vi "RPC Method MeasurementService Measure Logic.vi"(8 "error in":errorcluster, 11 "gRPCid in":T1) -> (0 "error out":errorcluster)   [LabVIEW 2020, in "MeasurementLink Measurement Server.lvlib"]
uses:
  MeasurementLink Measurement Server.lvlib
  <vilib>/gRPC/LabVIEW gRPC Library/Shared/grpcId.ctl
  Measurement Configuration.ctl
  <vilib>/gRPC/LabVIEW gRPC Library/Server API/typeDefs/gRPC Status Code.ctl
  6e93e594-9b53-4a41-bad0-565312cbf1e4.vi
  c01dd925-8d21-4ce6-b452-e7218c44af5c.vi
  <vilib>/gRPC/LabVIEW gRPC Library/Server API/Translate Protobuf Error.vi
  <vilib>/AdvancedString/1D String Array to Delimited String.vi
  <vilib>/gRPC/LabVIEW gRPC Library/Server API/Server/Get Server DLL Path.vi
  MeasurementContext/MeasurementContext.lvclass
  <vilib>/gRPC/LabVIEW gRPC Library/grpc-lvsupport-release.lvlib
  MeasurementLink Measurement Server Internal/RPC Service/MeasurementService/MeasurementService.lvclass
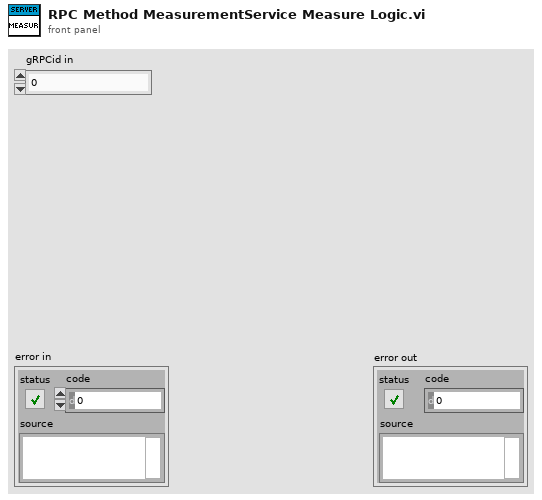
[diagram p1: front panel]
types:
  T1 = typedef "grpc-lvsupport-release.lvlib/grpcId.ctl" = u64
  T2 = typedef "MeasurementLink Measurement Server.lvlib/Measurement Configuration.ctl" = cluster{"Array in":dbl[]}
  T3 = typedef "MeasurementLink Measurement Server Internal.lvlib/ni_measurementlink_measurement_v1_MeasureRequest.ctl" = cluster{"configuration_parameters":T4, "pin_map_context":T5}
  T4 = typedef "MeasurementLink Measurement Server Internal.lvlib/google_protobuf_Any.ctl" = cluster{"type_url":string, "value":u8[]}
  T5 = typedef "MeasurementLink Measurement Server Internal.lvlib/ni_measurementlink_PinMapContext.ctl" = cluster{"pin_map_id":string, "sites":i32[]}
  T6 = typedef "MeasurementLink Measurement Server.lvlib/Measurement Results.ctl" = cluster{"Array out":dbl[]}
  T7 = typedef "grpc-lvsupport-release.lvlib/gRPC Status Code.ctl" = enum16{"OK", "CANCELLED", "UNKNOWN", "INVALID_ARGUMENT", "DEADLINE_EXCEEDED", "NOT_FOUND", "ALREADY_EXISTS", "PERMISSION_DENIED", "RESOURCE_EXHAUSTED", "FAILED_PRECONDITION", "ABORTED", "OUT_OF_RANGE", "UNIMPLEMENTED", "INTERNAL", "UNAVAILABLE", "DATA_LOSS", "UNAUTHENTICATED"}
  T8 = typedef "grpc-lvsupport-release.lvlib/Any.ctl" = cluster{"Type Url":string, "Bytes":u8[]}
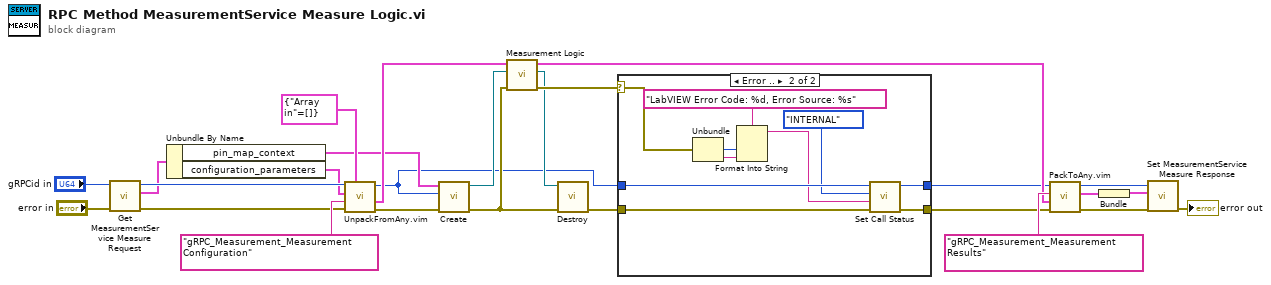
[diagram p0: block diagram]
diagram:
  n1 = call "Get MeasurementService Measure Request.vi"("error in (no error)"="error in", "gRPCid in"="gRPCid in") -> ("error out"=w9:errorcluster, "Message Data"=w10:T3, "gRPCid out"=w11:T1)  [unwired: 7 in]
  n2 = Unbundle By Name(w10) -> ("pin_map_context"=w5:T5, "configuration_parameters"=w6:T4)
  n3 = call "UnpackFromAny.vim"("Data Type"=T2 {"Array in"=[]} ("Measurement Configuration"), "error in"=w9, "Message Type"="gRPC_Measurement_Measurement Configuration", "Any"=w6, "gRPCid in"=w11) -> ("error out"=w7:errorcluster, "Unpacked Value"=w23:T2, "gRPCid out"=w1:u64)  [unwired: 4 in]
  n4 = call "Create.vi"("error in (no error)"=w7, "gRPC server call"=w1, "pin map context"=w5) -> ("error out"=w4:errorcluster, "MeasurementContext out"=w8:refnum<class "MeasurementContext.lvclass">)  [unwired: 7 in]
  n5 = call "Measurement Logic.vi"("error in"=w4, "Measurement Context"=w8, "Measurement Configuration"=w23) -> ("error out"=w17:errorcluster, "Measurement Context out"=w3:refnum<class "MeasurementContext.lvclass">, "Measurement Results"=w24:T6)  [unwired: 6 in]
  n6 = call-dynamic "Destroy.vi"("error in (no error)"=w4, "MeasurementContext in"=w3) -> ("error out"=w2:errorcluster)  [unwired: 9 in]
  n7 = case shown="Error .." w17 {
    selector: w17 -> [_ w38]
    tunnel: w1 -> [w28 w37]
    tunnel: [w28 w36] -> w16
    tunnel: w2 -> [w27 w34]
    tunnel: [w27 w35] -> w15
    frame No Error {
    }
    frame Error {
      n8 = Unbundle(w38) -> ("code"=w32:i32, "source"=w31:string)  [unwired: 1 out]
      n9 = Format Into String(format string="LabVIEW Error Code: %d, Error Source: %s", w32, w31) -> (resulting string=w29:string)  [unwired: 2 in, 1 out]
      n10 = call <vilib>:"Set Call Status.vi"("error in"=w34, "Details"=w29, "Status Code"=gRPC_Status_Code."INTERNAL", "gRPCid in"=w37) -> ("error out"=w35:errorcluster, "gRPCid out"=w36:T1)  [unwired: 6 in]
    }
  }
  n11 = call "PackToAny.vim"("error in"=w15, "Data To Pack"=w24, "Message Type"="gRPC_Measurement_Measurement Results", "gRPCid in"=w16) -> ("error out"=w18:errorcluster, "Any"=w20:T8, "gRPCid out"=w21:u64)  [unwired: 5 in]
  n12 = Bundle("Any"=w20) -> (w19:cluster{"Any":T8})  [unwired: 1 in]
  n13 = call "Set MeasurementService Measure Response.vi"("error in (no error)"=w18, "Message Data"=w19, "gRPCid in"=w21) -> ("error out"=→"error out":errorcluster)  [unwired: 8 in]
